vi "AIT - Utility - CRC - CRC.vi"(0 "Data String":string, 2 "Data Array":u8[](array[numeric]) format="0x%02x", 5 "error in (no error)":errorcluster, 7 "CRC Parameters":T1 {"Final CRC XOR Value" format="%.0x"; "Initial CRC Value" format="%.0x"; "CRC Polynomial" format="%.0x"}, 9 "CRC Calculation":T2) -> (14 "CRC (U32)":u32 format="%.0x", 16 "CRC (U16)":u16 format="%.0x", 18 "CRC (U8)":u8 format="%.0x", 19 "error out":errorcluster)   [LabVIEW 2020, in "Library Commun.lvlib"]
uses:
  Library Commun.lvlib
  Support/AIT - Utility - CRC - CRC Type.ctl
  Support/AIT - Utility - CRC - CRC Parameters.ctl
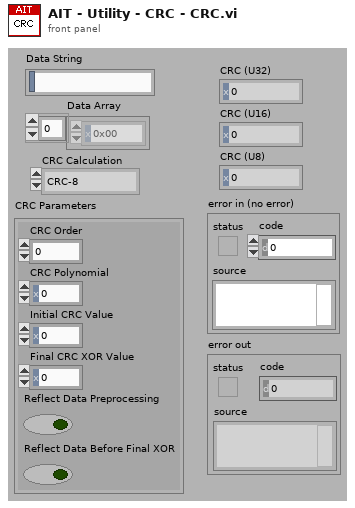
[diagram p1: front panel]
types:
  T1 = typedef "Library Commun.lvlib/AIT - Utility - CRC - CRC Parameters.ctl" = cluster{"CRC Order":u8, "CRC Polynomial":u32, "Initial CRC Value":u32, "Final CRC XOR Value":u32, "Reflect Data Preprocessing":bool, "Reflect Data Before Final XOR":bool}
  T2 = typedef "Library Commun.lvlib/AIT - Utility - CRC - CRC Type.ctl" = enum16{"CRC-8", "CRC-16", "CRC-32", "CRC-CCITT", "Other (specify)"}
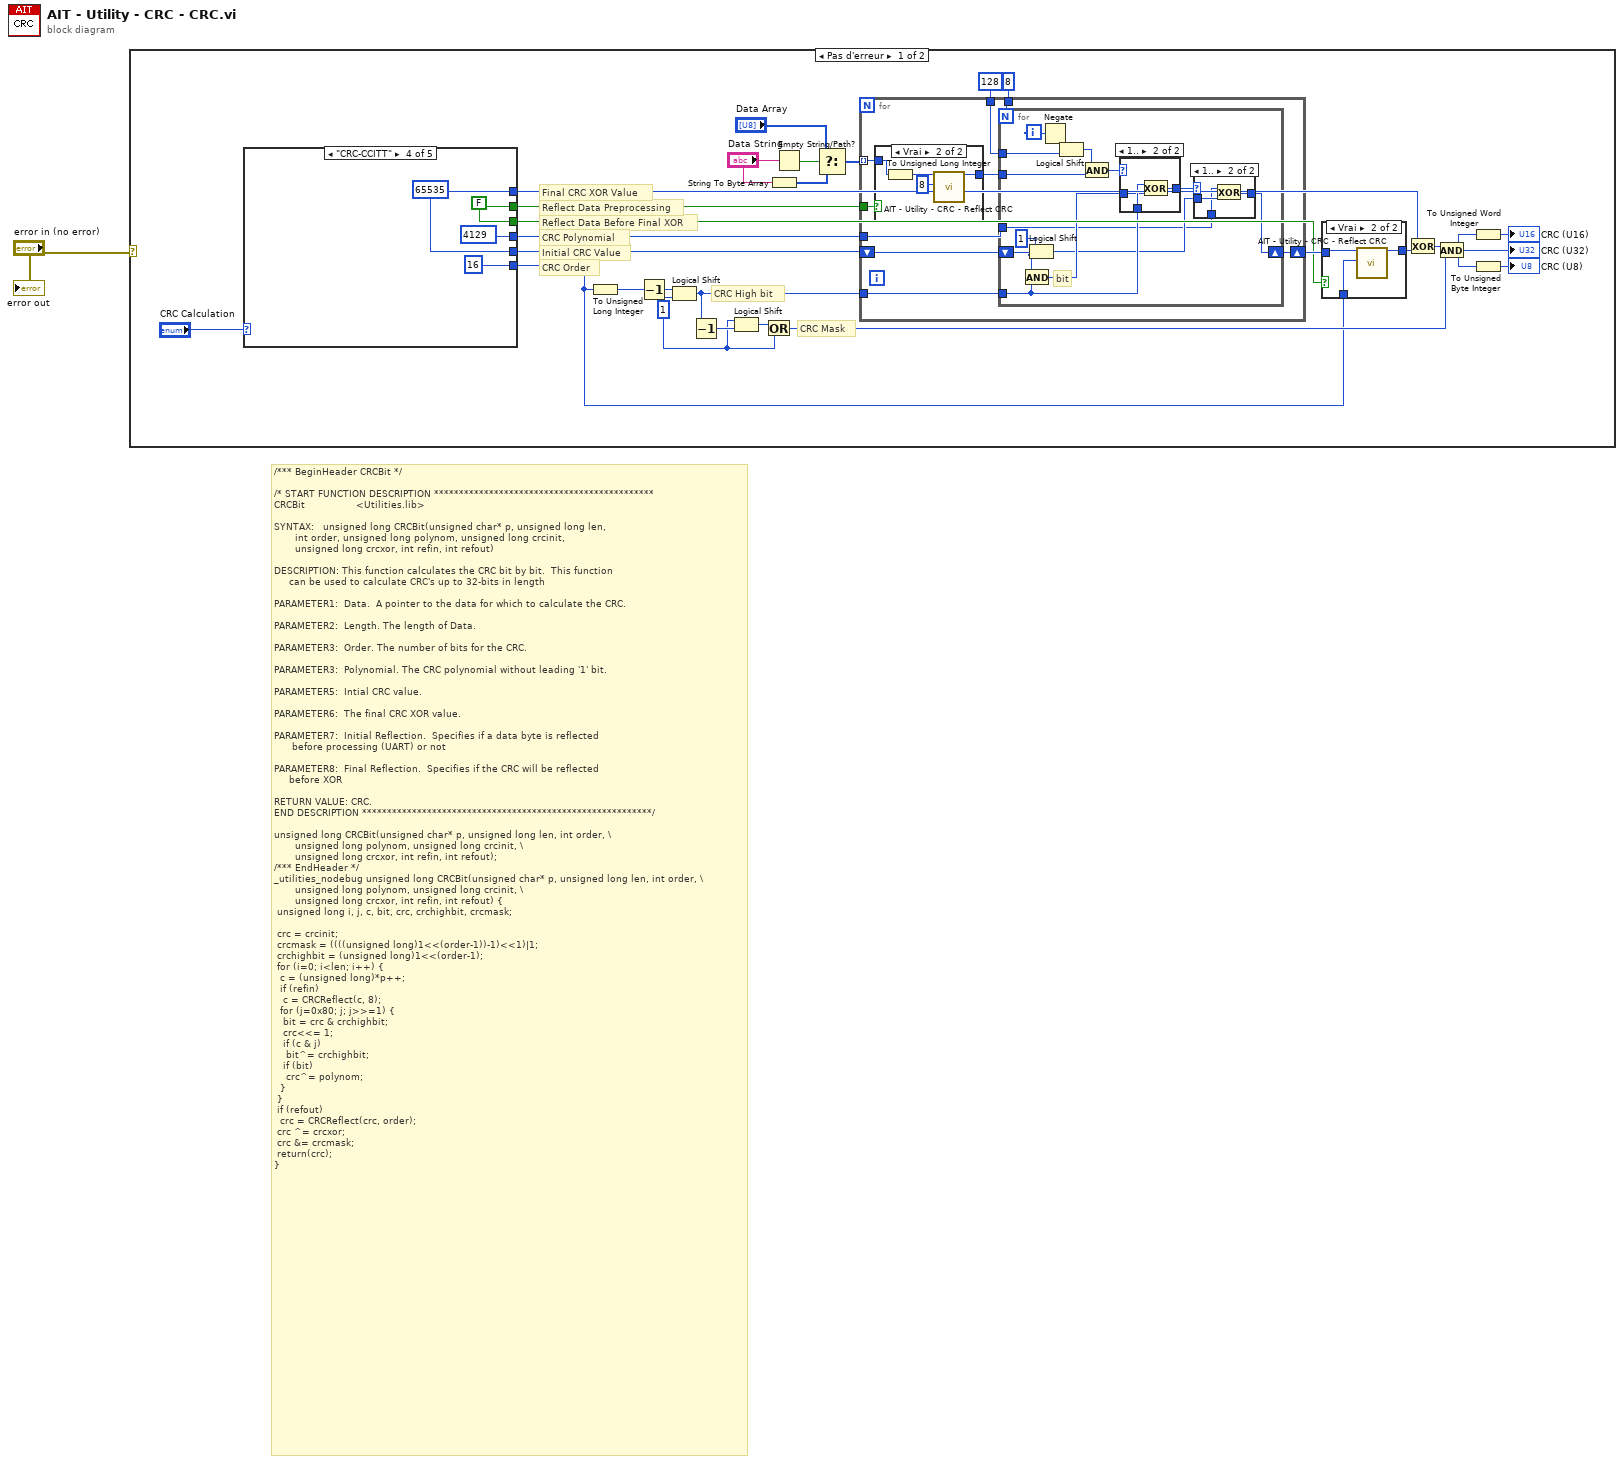
[diagram p0: block diagram]
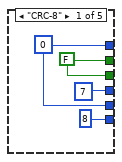
[diagram p6: hidden frame]
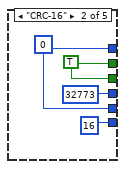
[diagram p7: hidden frame]
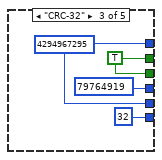
[diagram p8: hidden frame]
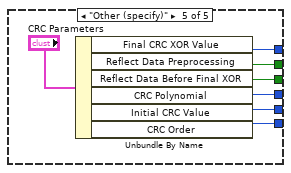
[diagram p9: hidden frame]
diagram:
  # "/*** BeginHeader CRCBit */\n\n/* START FUNCTION DESCRIPTION ********************************************\nCRCBit\t\t\t\t\t\t\t\t\t\t\t\t\t\t\t\t\t<Utilities.lib>\n\nSYNTAX:\t\t\tunsigned long CRCBit(unsigned char* p, unsigned long len,\n\t\t\t\t\t\t\tint order, unsigned long polynom, unsigned long crcinit,\n\t\t\t\t\t\t\tunsigned long crcxor, int refin, int refout)\n\nDESCRIPTION:\tThis function calculates the CRC bit by bit.  This function\n\t\t\t\t\tcan be used to calculate CRC's up to 32-bits in length\n\nPARAMETER1:\t\tData.  A pointer to the data for which to calculate the CRC.\n\nPARAMETER2:\t\tLength.\tThe length of Data.\n\nPARAMETER3:\t\tOrder.\tThe number of bits for the CRC.\n\nPARAMETER3:\t\tPolynomial.\tThe CRC polynomial without leading '1' bit.\n\nPARAMETER5:\t\tIntial CRC value.\n\nPARAMETER6:\t\tThe final CRC XOR value.\n\nPARAMETER7:\t\tInitial Reflection.  Specifies if a data byte is reflected\n\t\t\t\t\t\tbefore processing (UART) or not\n\nPARAMETER8:\t\tFinal Reflection.  Specifies if the CRC will be reflected\n\t\t\t\t\tbefore XOR\n\nRETURN VALUE:\tCRC.\nEND DESCRIPTION **********************************************************/\n\nunsigned long CRCBit(unsigned char* p, unsigned long len, int order, \\\n\t\t\t\t\t\t\tunsigned long polynom, unsigned long crcinit, \\\n\t\t\t\t\t\t\tunsigned long crcxor, int refin, int refout);\n/*** EndHeader */\n_utilities_nodebug unsigned long CRCBit(unsigned char* p, unsigned long len, int order, \\\n\t\t\t\t\t\t\tunsigned long polynom, unsigned long crcinit, \\\n\t\t\t\t\t\t\tunsigned long crcxor, int refin, int refout) {\n\tunsigned long i, j, c, bit, crc, crchighbit, crcmask;\n\n\tcrc = crcinit;\n\tcrcmask = ((((unsigned long)1<<(order-1))-1)<<1)|1;\n\tcrchighbit = (unsigned long)1<<(order-1);\n\tfor (i=0; i<len; i++) {\n\t\tc = (unsigned long)*p++;\n\t\tif (refin)\n\t\t\tc = CRCReflect(c, 8);\n\t\tfor (j=0x80; j; j>>=1) {\n\t\t\tbit = crc & crchighbit;\n\t\t\tcrc<<= 1;\n\t\t\tif (c & j)\n\t\t\t\tbit^= crchighbit;\n\t\t\tif (bit)\n\t\t\t\tcrc^= polynom;\n\t\t}\n\t}\t\n\tif (refout)\n\t\tcrc = CRCReflect(crc, order);\n\tcrc ^= crcxor;\n\tcrc &= crcmask;\n\treturn(crc);\n}"
  n1 = case shown="Pas d'erreur" "error in (no error)" {
    frame No Error {
      w23 = u32 1 ("x")
      # "CRC Order"
      # "Initial CRC Value"
      # "CRC Polynomial"
      # "Reflect Data Before Final XOR"
      # "Reflect Data Preprocessing"
      # "Final CRC XOR Value"
      # "CRC Mask"
      # "CRC High bit"
      n2 = case shown="\"CRC-CCITT\"" "CRC Calculation" {
        tunnel: [w70 w75 w80 w83 w91] -> w7
        tunnel: [w69 w73 w77 w81 w89] -> w6
        tunnel: [w69 w73 w77 w81 w90] -> w5
        tunnel: [u32 7 ("CRC Polynomial") u32 32773 ("CRC Polynomial") u32 79764919 ("CRC Polynomial") u32 4129 ("CRC Polynomial") w88] -> w4
        tunnel: [w70 w75 w80 w83 w86] -> w3
        tunnel: [u8 8 ("CRC Order") u8 16 ("CRC Order") u8 32 ("CRC Order") u8 16 ("CRC Order") w87] -> w2
        frame "CRC-8" {
          w69 = FALSE ("Reflect Data Preprocessing")
          w70 = u32 0 ("Initial CRC Value")
        }
        frame "CRC-16" {
          w73 = TRUE ("Reflect Data Preprocessing")
          w75 = u32 0 ("Initial CRC Value")
        }
        frame "CRC-32" {
          w77 = TRUE ("Reflect Data Preprocessing")
          w80 = u32 4294967295 ("Initial CRC Value")
        }
        frame "CRC-CCITT" {
          w81 = FALSE ("Reflect Data Preprocessing")
          w83 = u32 65535 ("Initial CRC Value")
        }
        frame "Other (specify)" {
          n3 = Unbundle By Name("CRC Parameters") -> ("Final CRC XOR Value"=w91:u32, "Reflect Data Preprocessing"=w89:bool, "Reflect Data Before Final XOR"=w90:bool, "CRC Polynomial"=w88:u32, "Initial CRC Value"=w86:u32, "CRC Order"=w87:u8)
        }
      }
      n4 = To Unsigned Long Integer(number=w2) -> (unsigned 32bit integer=w11:u32)
      n5 = Decrement(x=w11) -> (x-1=w27:u32)
      n6 = Logical Shift(y=w27, x=w23) -> (x << y=w26:u32)
      n7 = Decrement(x=w26) -> (x-1=w25:u32)
      n8 = Logical Shift(y=w23, x=w25) -> (x << y=w24:u32)
      n9 = Or(x=w24, y=w23) -> (x .or. y?=w12:u32)
      n10 = String To Byte Array(string="Data String") -> (unsigned byte array=w22:u8[])
      n11 = Empty String/Path?(string/path="Data String") -> (empty?=w19:bool)
      n12 = Select(t="Data Array", s=w19, f=w22) -> (s? t:f=w18:u8[])
      n13 = for {
        shift-right: [w34] -> w15
        shift-left: w3 -> [w39]
        tunnel: w26 -> [w38]
        tunnel: w18 -> [w33] mode=indexing
        tunnel: w6 -> [w41]
        tunnel: u8 8 ("Bits") -> [w40]
        tunnel: u32 128 -> [w37]
        tunnel: w4 -> [w35]
        n14 = case shown="Vrai" w41 {
          tunnel: [w64 w67] -> w36
          tunnel: w33 -> [w64 w66]
          frame False {
          }
          frame True {
            n15 = To Unsigned Long Integer(number=w66) -> (unsigned 32bit integer=w65:u32)
            n16 = call "AIT - Utility - CRC - Reflect CRC.vi"("CRC"=w65, "Bits"=u8 8) -> ("Reflected CRC"=w67:u32)  [unwired: 16 in, 1 out]
          }
        }
        n17 = for {
          N: w40 -> [_]
          shift-right: [w42] -> w34
          shift-left: w39 -> [w55]
          tunnel: w38 -> [w48]
          tunnel: w37 -> [w53]
          tunnel: w36 -> [w52]
          tunnel: w35 -> [w45]
          i -> [w44]
          # "bit"
          n18 = And(x=w55, y=w48) -> (x .and. y?=w49:u32)
          n19 = Logical Shift(y=u32 1, x=w55) -> (x << y=w46:u32)
          n20 = Negate(x=w44) -> (-x=w43:i32)
          n21 = Logical Shift(y=w43, x=w53) -> (x << y=w51:u32)
          n22 = And(x=w51, y=w52) -> (x .and. y?=w50:u32)
          n23 = case shown="1.." w50 {
            tunnel: w49 -> [w60 w61]
            tunnel: [w60 w63] -> w47
            tunnel: w48 -> [_ w62]
            frame ..0 {
            }
            frame 1.. {
              n24 = Exclusive Or(1:w61, 2:w62) -> (0:w63:u32)
            }
          }
          n25 = case shown="1.." w47 {
            tunnel: w46 -> [w56 w58]
            tunnel: [w56 w59] -> w42
            tunnel: w45 -> [_ w57]
            frame ..0 {
            }
            frame 1.. {
              n26 = Exclusive Or(1:w58, 2:w57) -> (0:w59:u32)
            }
          }
        }
      }
      n27 = case shown="Vrai" w5 {
        tunnel: w15 -> [w29 w32]
        tunnel: [w29 w31] -> w14
        tunnel: w2 -> [_ w30]
        frame False {
        }
        frame True {
          n28 = call "AIT - Utility - CRC - Reflect CRC.vi"("CRC"=w32, "Bits"=w30) -> ("Reflected CRC"=w31:u32)  [unwired: 16 in, 1 out]
        }
      }
      n29 = Exclusive Or(1:w14, 2:w7) -> (0:w13:u32)
      n30 = And(x=w13, y=w12) -> (x .and. y?=w10:u32)
      "CRC (U32)" <- w10
      n31 = To Unsigned Word Integer(number=w10) -> (unsigned 16bit integer=→"CRC (U16)":u16)
      n32 = To Unsigned Byte Integer(number=w10) -> (unsigned 8bit integer=→"CRC (U8)":u8)
    }
    frame Error {
    }
  }
  "error out" <- "error in (no error)"
